vi "Q_Get Total Distance in KM by Athlete split by Type.vi"(8 "error in (no error)":errorcluster, 11 "Data Manager in":refnum<class "Data Manager.lvclass">) -> (0 "error out":errorcluster, 1 "Run":string[][](table), 2 "Walk":string[][](table), 3 "Data Manager out":refnum<class "Data Manager.lvclass">, 4 "Ride":string[][](table))   [LabVIEW 2020, in "Data Manager.lvclass"]
uses:
  Data Manager.lvclass
  Data Manager.lvclass/Data Manager.ctl
  <vilib>/drjdpowell/SQLite Library/SQL Connection/Execute SQL.vi
  <vilib>/drjdpowell/SQLite Library/SQLite.lvlib
  <vilib>/drjdpowell/SQLite Library/SQL Connection/Connection.lvclass
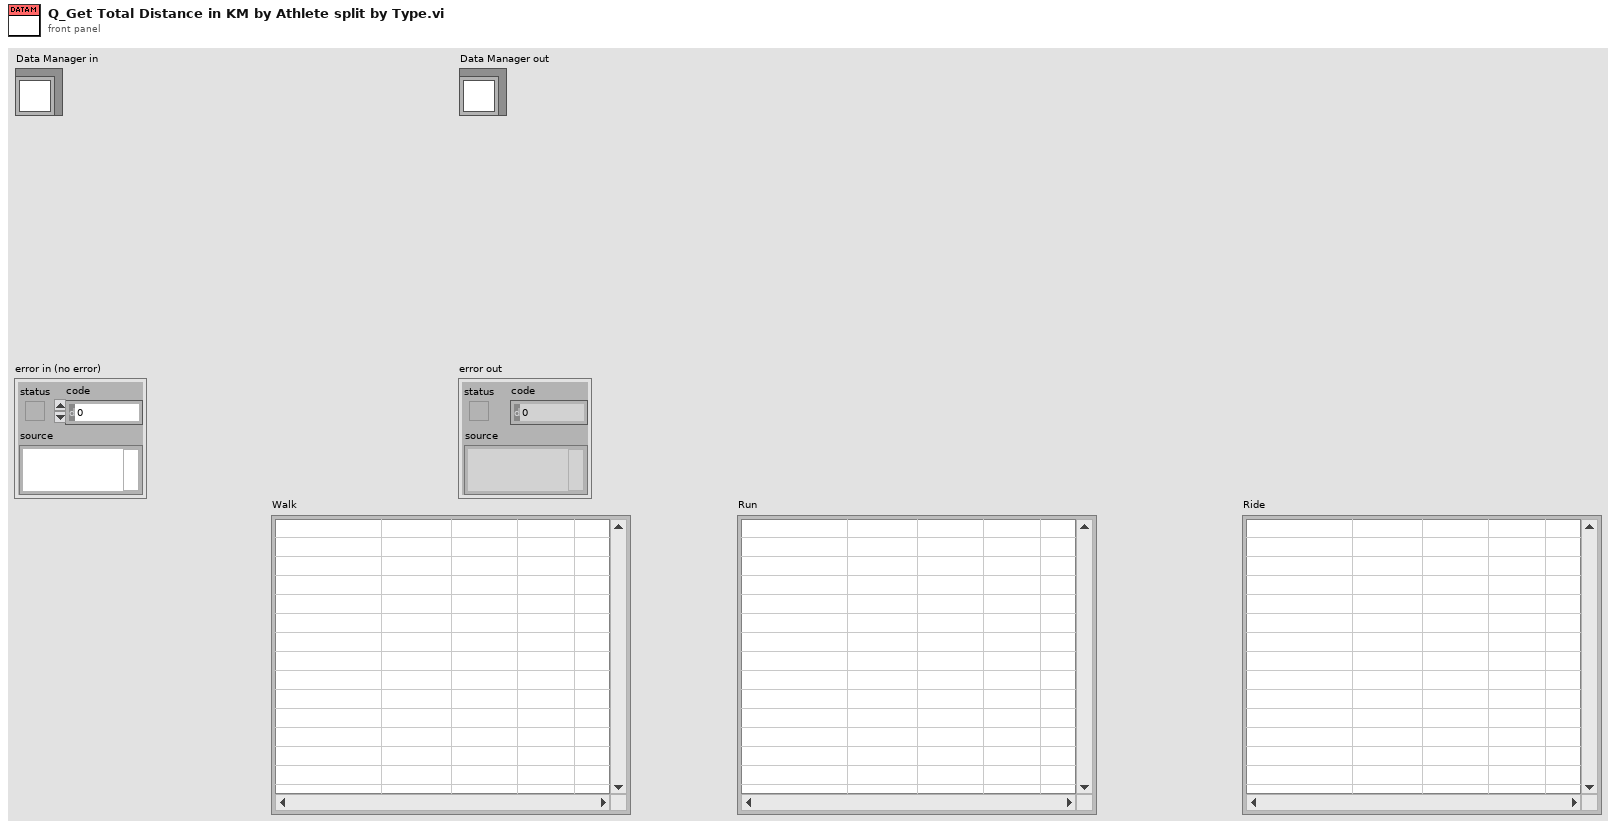
[diagram p1: front panel]
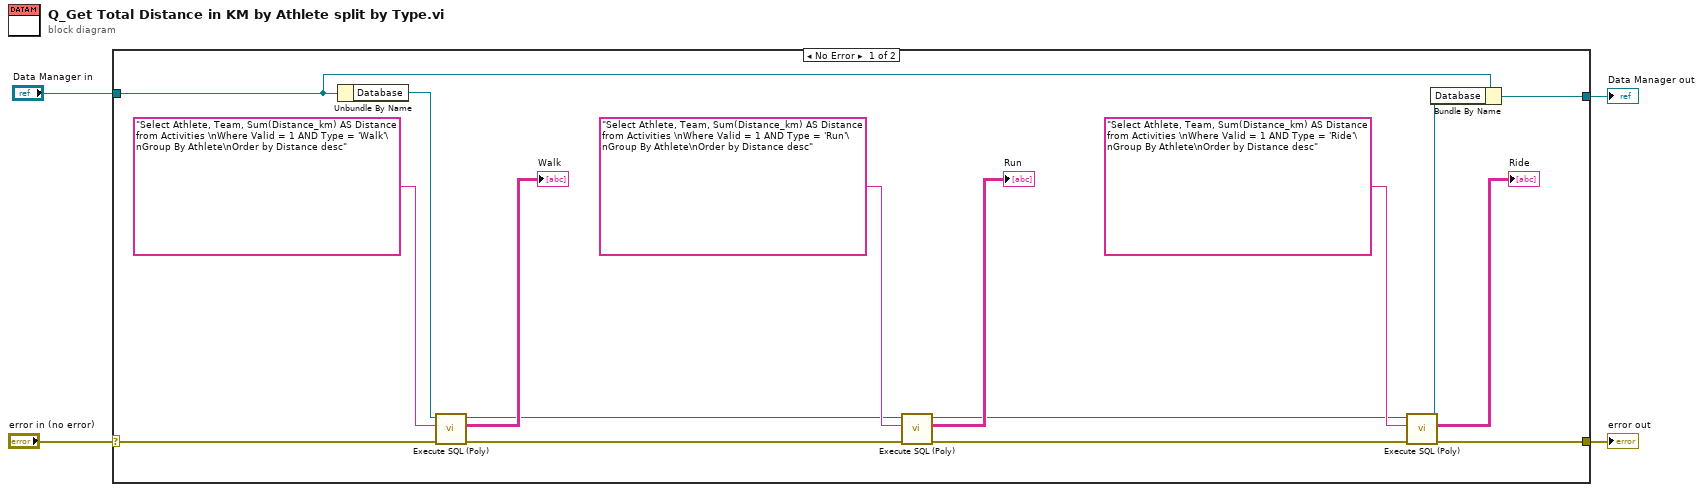
[diagram p0: block diagram]
diagram:
  n1 = case shown="No Error" "error in (no error)" {
    selector: "error in (no error)" -> [w17 w22]
    tunnel: [w5 w22] -> w3
    tunnel: [w18 w21] -> w1
    tunnel: "Data Manager in" -> [w19 w21]
    frame No Error {
      n2 = Unbundle By Name(w19) -> ("Database"=w20:refnum<class "Connection.lvclass">)
      n3 = call-poly <vilib>:"Execute SQL (Poly).vi"("error in (no error)"=w17, "SQL"="Select Athlete, Team, Sum(Distance_km) AS Distance from Activities \nWhere Valid = 1 AND Type = 'Walk'\nGroup By Athlete\nOrder by Distance desc", "SQLite Connection in"=w20) -> ("error out"=w7:errorcluster, "Result Set"=→"Walk":string[][], "SQLite Connection"=w8:refnum<class "Connection.lvclass">)  [unwired: 5 in, 1 out]
      n4 = call-poly <vilib>:"Execute SQL (Poly).vi"("error in (no error)"=w7, "SQL"="Select Athlete, Team, Sum(Distance_km) AS Distance from Activities \nWhere Valid = 1 AND Type = 'Run'\nGroup By Athlete\nOrder by Distance desc", "SQLite Connection in"=w8) -> ("error out"=w6:errorcluster, "Result Set"=→"Run":string[][], "SQLite Connection"=w9:refnum<class "Connection.lvclass">)  [unwired: 5 in, 1 out]
      n5 = call-poly <vilib>:"Execute SQL (Poly).vi"("error in (no error)"=w6, "SQL"="Select Athlete, Team, Sum(Distance_km) AS Distance from Activities \nWhere Valid = 1 AND Type = 'Ride'\nGroup By Athlete\nOrder by Distance desc", "SQLite Connection in"=w9) -> ("error out"=w5:errorcluster, "Result Set"=→"Ride":string[][], "SQLite Connection"=w10:refnum<class "Connection.lvclass">)  [unwired: 5 in, 1 out]
      n6 = Bundle By Name(cluster=w19, "Database"=w10) -> (w18:refnum<class "Data Manager.lvclass">)
    }
    frame Error {
    }
  }
  "error out" <- w3
  "Data Manager out" <- w1
